vi "Ctx Set.vi"(7 "path override":path, 8 "error in (no error)":errorcluster, 9 "optval_":i32, 10 "option_":i32, 11 "context_":u32) -> (0 "error out":errorcluster, 3 "context_ out":u32)   [LabVIEW 2025, in "LibZMQ.lvlib"]
doc: "ZMQ_EXPORT int zmq_ctx_set (void *context_, int option_, int optval_);"
uses:
  LibZMQ.lvlib
  errno.vi
  strerror.vi
  <vilib>/Utility/error.llb/Error Cluster From Error Code.vi
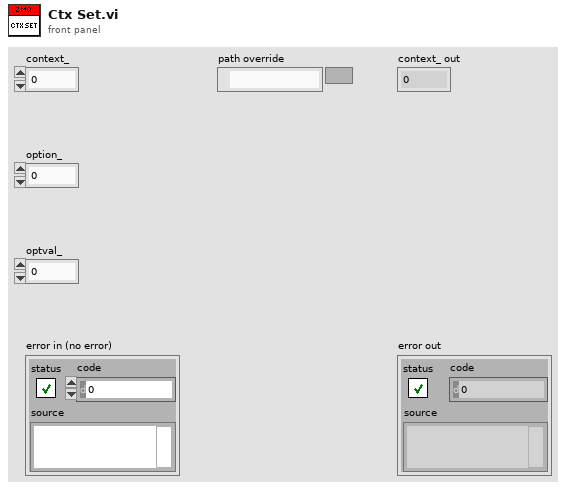
[diagram p1: front panel]
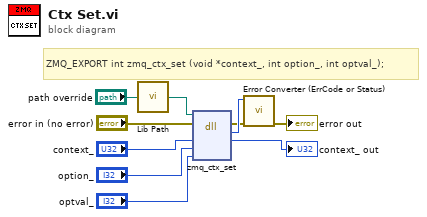
[diagram p0: block diagram]
diagram:
  # "ZMQ_EXPORT int zmq_ctx_set (void *context_, int option_, int optval_);"
  n1 = call "Lib Path.vi"("path override"="path override") -> ("lib path"=w1:path)
  n2 = dll-call lib="C:/git/ZA/libzmq-v143-mt-4_3_6/lib/win32/libzmq-v143-mt-4_3_6.*" fn="zmq_ctx_set"(path in=w1, error in="error in (no error)", "context_"="context_", "option_"="option_", "optval_"="optval_") -> (error out=w4:errorcluster, "return type"=w10:i32, "context_"=→"context_ out":u32)  [unwired: 3 in, 1 out]
  n3 = call "Error Converter (ErrCode or Status).vi"("error in (no error)"=w4, "error code"=w10) -> ("error out"=→"error out":errorcluster)  [unwired: 9 in]
